vi "Movie File Suffix.vi"(9 "Movie Series In":T1={"Fields"=1, "Lanes"=1, "Acquisition type"=enum."Movie series", "Sweeps"=[]}, 11 "Base Path In":path) -> (3 "Base Paths":path[](array[path]))   [LabVIEW 2023, in "Automation.lvlib"]
uses:
  Resources/Type Defs/Movie Series.ctl
  Resources/Type Defs/Movie auto-numbering.ctl
  Resources/Type Defs/Param Sweep.ctl
  Resources/Type Defs/Sweep Parameter.ctl
  Automation.lvlib
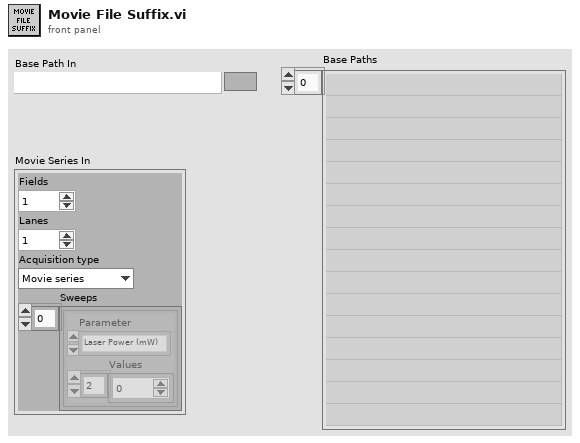
[diagram p1: front panel]
types:
  T1 = typedef "Movie Series.ctl" = cluster{"Fields":i32, "Lanes":i32, "Acquisition type":T2, "Sweeps":T3[]}
  T2 = typedef "Movie auto-numbering.ctl" = enum16{"Single movie", "Movie series", "Multi-lane series", "Sweep Parameter"}
  T3 = typedef "Param Sweep.ctl" = cluster{"Parameter":T4, "Values":u32[]}
  T4 = typedef "Sweep Parameter.ctl" = enum16{"Laser Power (mW)", "Exposure Time (ms)", "Number of Frames", "Laser Line (1,2,3,4)"}
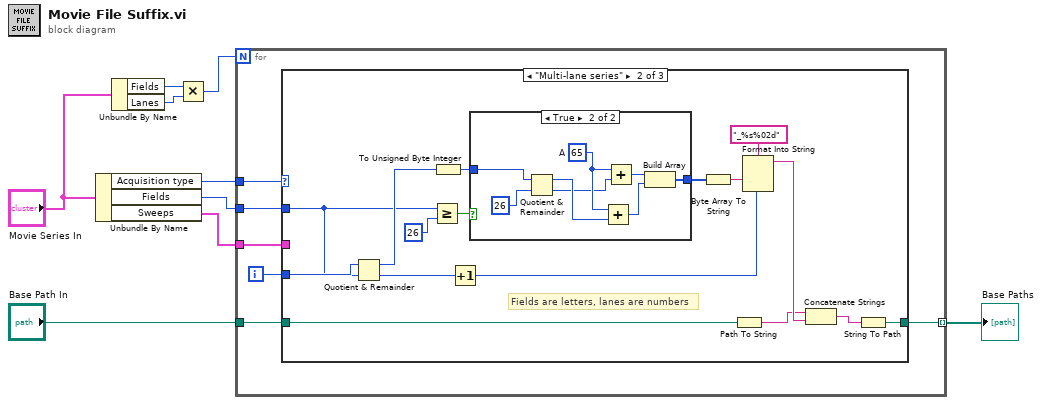
[diagram p0: block diagram]
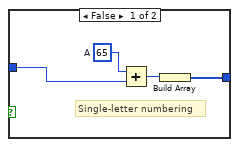
[diagram p3: hidden frame]
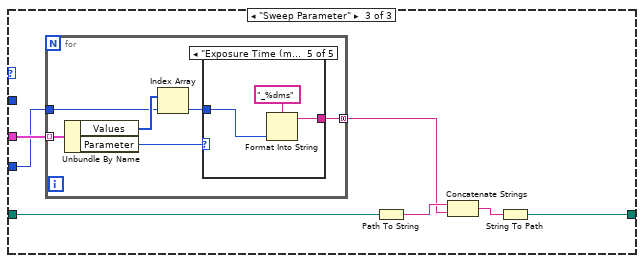
[diagram p4: hidden frame]
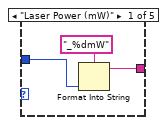
[diagram p5: hidden frame]
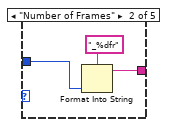
[diagram p6: hidden frame]
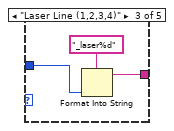
[diagram p7: hidden frame]
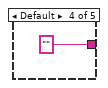
[diagram p8: hidden frame]
diagram:
  n1 = Unbundle By Name("Movie Series In") -> ("Acquisition type"=w4:T2, "Fields"=w3:i32, "Sweeps"=w2:T3[])
  n2 = Unbundle By Name("Movie Series In") -> ("Fields"=w7:i32, "Lanes"=w6:i32)
  n3 = Multiply(x=w7, y=w6) -> (x*y=w5:i32)
  n4 = for {
    N: w5 -> [_]
    tunnel: "Base Path In" -> [w14]
    tunnel: [w15] -> w1 mode=indexing
    tunnel: w4 -> [w12]
    tunnel: w3 -> [w11]
    tunnel: w2 -> [w10]
    i -> [w13]
    n5 = case shown="\"Multi-lane series\"" w12 {
      tunnel: [w16 w18 w45] -> w15
      tunnel: w14 -> [w16 w19 w46]
      tunnel: w13 -> [_ w32 w50]
      tunnel: w11 -> [_ w22 _]
      tunnel: w10 -> [_ _ w51]
      frame Default {
      }
      frame "Multi-lane series" {
        # "Fields are letters, lanes are numbers"
        n6 = Quotient & Remainder(x=w32, y=w22) -> (x-y*floor(x/y)=w25:i32, floor(x/y)=w30:i32)
        n7 = Greater Or Equal?(x=w22, y=u8 26) -> (x >= y?=w27:bool)
        n8 = To Unsigned Byte Integer(number=w25) -> (unsigned 8bit integer=w24:u8)
        n9 = Increment(x=w30) -> (x+1=w29:i32)
        n10 = case shown="True" w27 {
          tunnel: [w33 w43] -> w28
          tunnel: w24 -> [w35 w42]
          frame False {
            w36 = u8 65  # A
            # "Single-letter numbering"
            n11 = Add(x=w36, y=w35) -> (x+y=w34:u8)
            n12 = Build Array(w34) -> (w33:u8[])
          }
          frame True {
            w40 = u8 65  # A
            n13 = Quotient & Remainder(x=w42, y=u8 26) -> (x-y*floor(x/y)=w38:u8, floor(x/y)=w37:u8)
            n14 = Add(x=w40, y=w38) -> (x+y=w39:u8)
            n15 = Add(x=w40, y=w37) -> (x+y=w44:u8)
            n16 = Build Array(w44, w39) -> (w43:u8[])
          }
        }
        n17 = Byte Array To String(unsigned byte array=w28) -> (string=w23:string)
        n18 = Path To String(path=w19) -> (string=w20:string)
        n19 = Format Into String(format string="_%s%02d", w23, w29) -> (resulting string=w21:string)  [unwired: 2 in, 1 out]
        n20 = Concatenate Strings(w20, w21) -> (w17:string)
        n21 = String To Path(string=w17) -> (path=w18:path)
      }
      frame "Sweep Parameter" {
        n22 = for {
          tunnel: [w52] -> w47 mode=concatenating
          tunnel: w51 -> [w57] mode=indexing
          tunnel: w50 -> [w54]
          n23 = Unbundle By Name(w57) -> ("Values"=w55:u32[], "Parameter"=w56:T4)
          n24 = Index Array(array=w55, index=w54) -> (element=w53:u32)
          n25 = case shown="\"Exposure Time (ms)\"" w56 {
            tunnel: [w59 w63 w65 "" w69] -> w52
            tunnel: w53 -> [w58 w61 w64 _ w70]
            frame "Laser Power (mW)" {
              n26 = Format Into String(format string="_%dmW", w58) -> (resulting string=w59:string)  [unwired: 2 in, 1 out]
            }
            frame "Number of Frames" {
              n27 = Format Into String(format string="_%dfr", w61) -> (resulting string=w63:string)  [unwired: 2 in, 1 out]
            }
            frame "Laser Line (1,2,3,4)" {
              n28 = Format Into String(format string="_laser%d", w64) -> (resulting string=w65:string)  [unwired: 2 in, 1 out]
            }
            frame Default {
            }
            frame "Exposure Time (ms)" {
              n29 = Format Into String(format string="_%dms", w70) -> (resulting string=w69:string)  [unwired: 2 in, 1 out]
            }
          }
        }
        n30 = Path To String(path=w46) -> (string=w49:string)
        n31 = Concatenate Strings(w49, w47) -> (w48:string)
        n32 = String To Path(string=w48) -> (path=w45:path)
      }
    }
  }
  "Base Paths" <- w1
